vi "Voltage Sweep Merge.vi"() -> ()   [LabVIEW 2017]
doc: "This example shows how to create, run a script and query the script output data."
uses:
  <vilib>/Utility/file.llb/Write Delimited Spreadsheet (string).vi
  <instrlib>/Keithley 2600 Series/Keithley 2600 Series.lvlib
panel:
  out "Graph 3":T1(graph)
  in  "Working Folder":path=path "~"
  out "PCE(a.u.)":dbl
  in  "Pin(W/cm^2)":dbl=0.1
  out "FF(a.u.)":dbl
  out "Jsc(A/cm^2)":dbl
  in  "Area(cm^2)":dbl=0.085
  out "Ioc(A)":dbl
  out "Voc(V)":dbl
  out "Vsc(V)":dbl
  out "Isc(A)":dbl
  out "IMP(A)":dbl
  out "VMP(V)":dbl
  out "PMP(W)":dbl
  out "output array":string[][](array[string])
  in  "SweepSetting":T2={"CurrentLimit(A)"=0.1, "Start Voltage(V)"=-0.5, "Stop Voltage(V)"=0.9, "Dwell Time(mS)"=150.0, "NumPoint"=75.0} {"NumPoint" min=1.0 max=75.0 step=1.0; "Dwell Time(mS)" min=50.0 max=150.0; "Stop Voltage(V)" min=-200.0 max=200.0; "Start Voltage(V)" min=-200.0 max=200.0; "CurrentLimit(A)" min=1e-09 max=1.5}
  out "Graph 2":T1(graph)
  out "Sweep":i32
  in  "Inter Sweep Delay(s)":dbl=1.0 min=0.1 max=3600.0
  out "Seconds":i32
  out "Minutes":i32
  out "Hours":i32
  in  "Stop Button":bool
  in  "Aperture State (Channel B)":u16(ring) items=["Always OFF", "Always ON", "ON During Sweep OFF Otherwise", "OFF During Sweep ON Otherwise"]
  in  "Number of Sweeps":dbl=3.0 min=1.0 max=1000.0 step=1.0
  in  "USB COM Port":refnum<visa-resource-name>="COM3"
  # "Time Remaining"
  # ":"
  # ":"
  # "Sweep Setting\n(Channel A)"
  # "2634B can output up to 20.2 V at 1.5 A,\n or 202 V at 100 mA current limit."
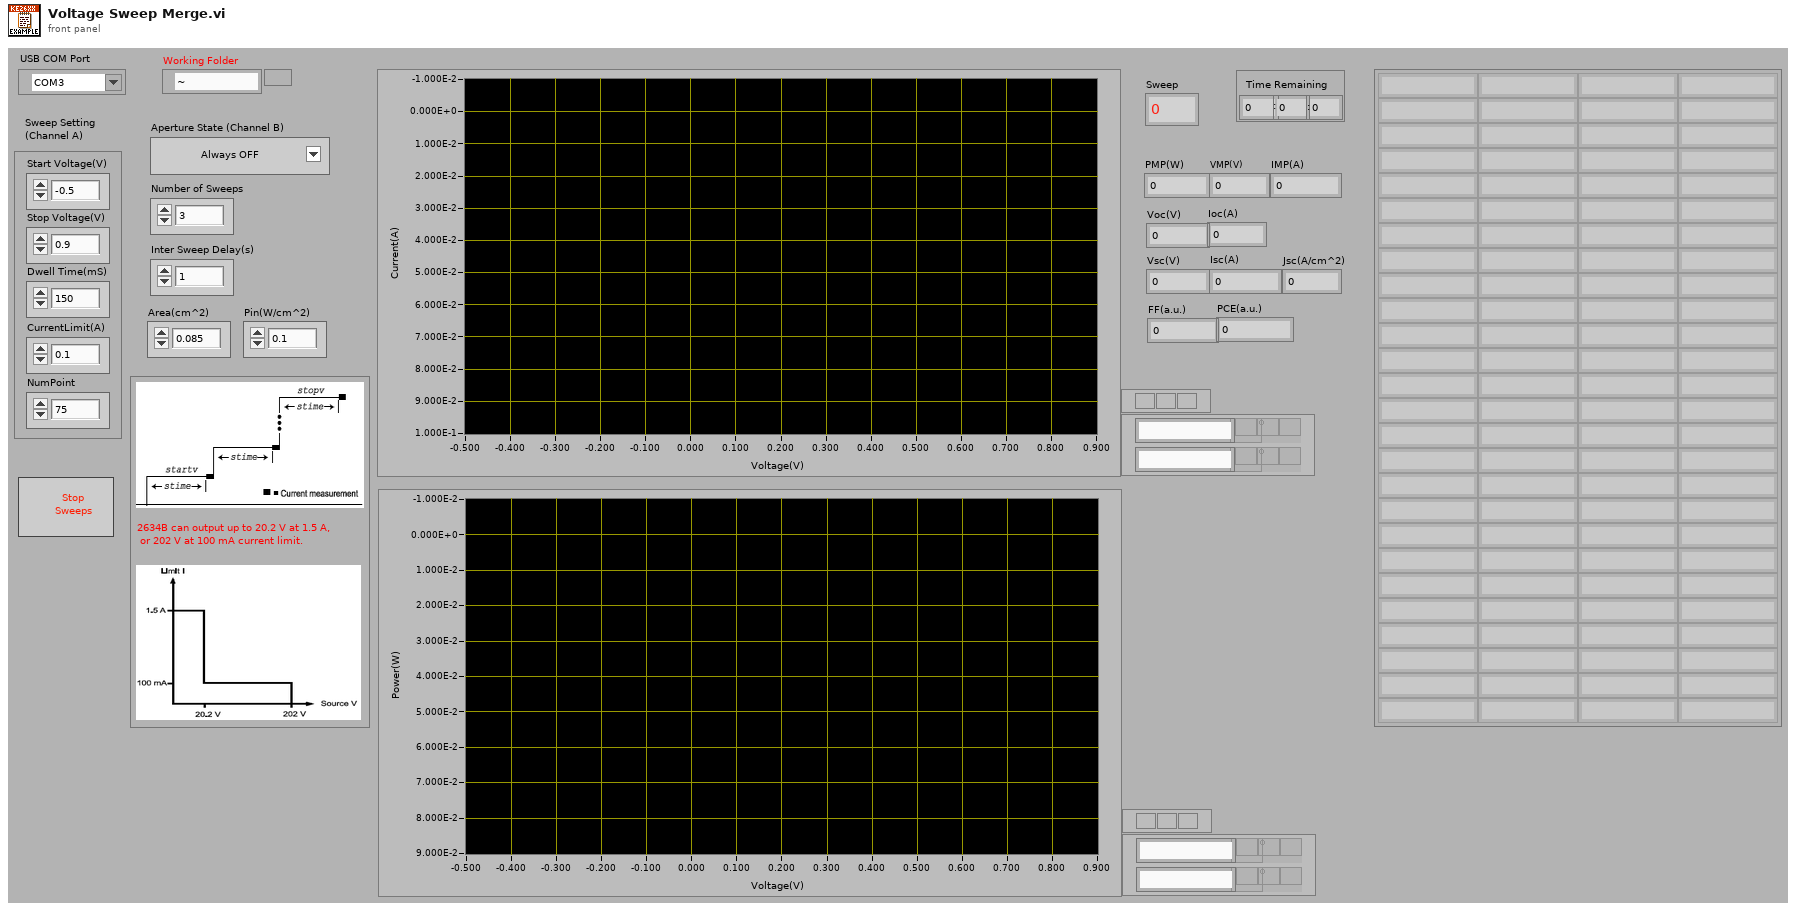
[diagram p1: front panel]
types:
  T1 = cluster{"array type (2D Dbl)":dbl[], "array type (2D Dbl)":dbl[]}
  T2 = cluster{"CurrentLimit(A)":dbl, "Start Voltage(V)":dbl, "Stop Voltage(V)":dbl, "Dwell Time(mS)":dbl, "NumPoint":dbl}
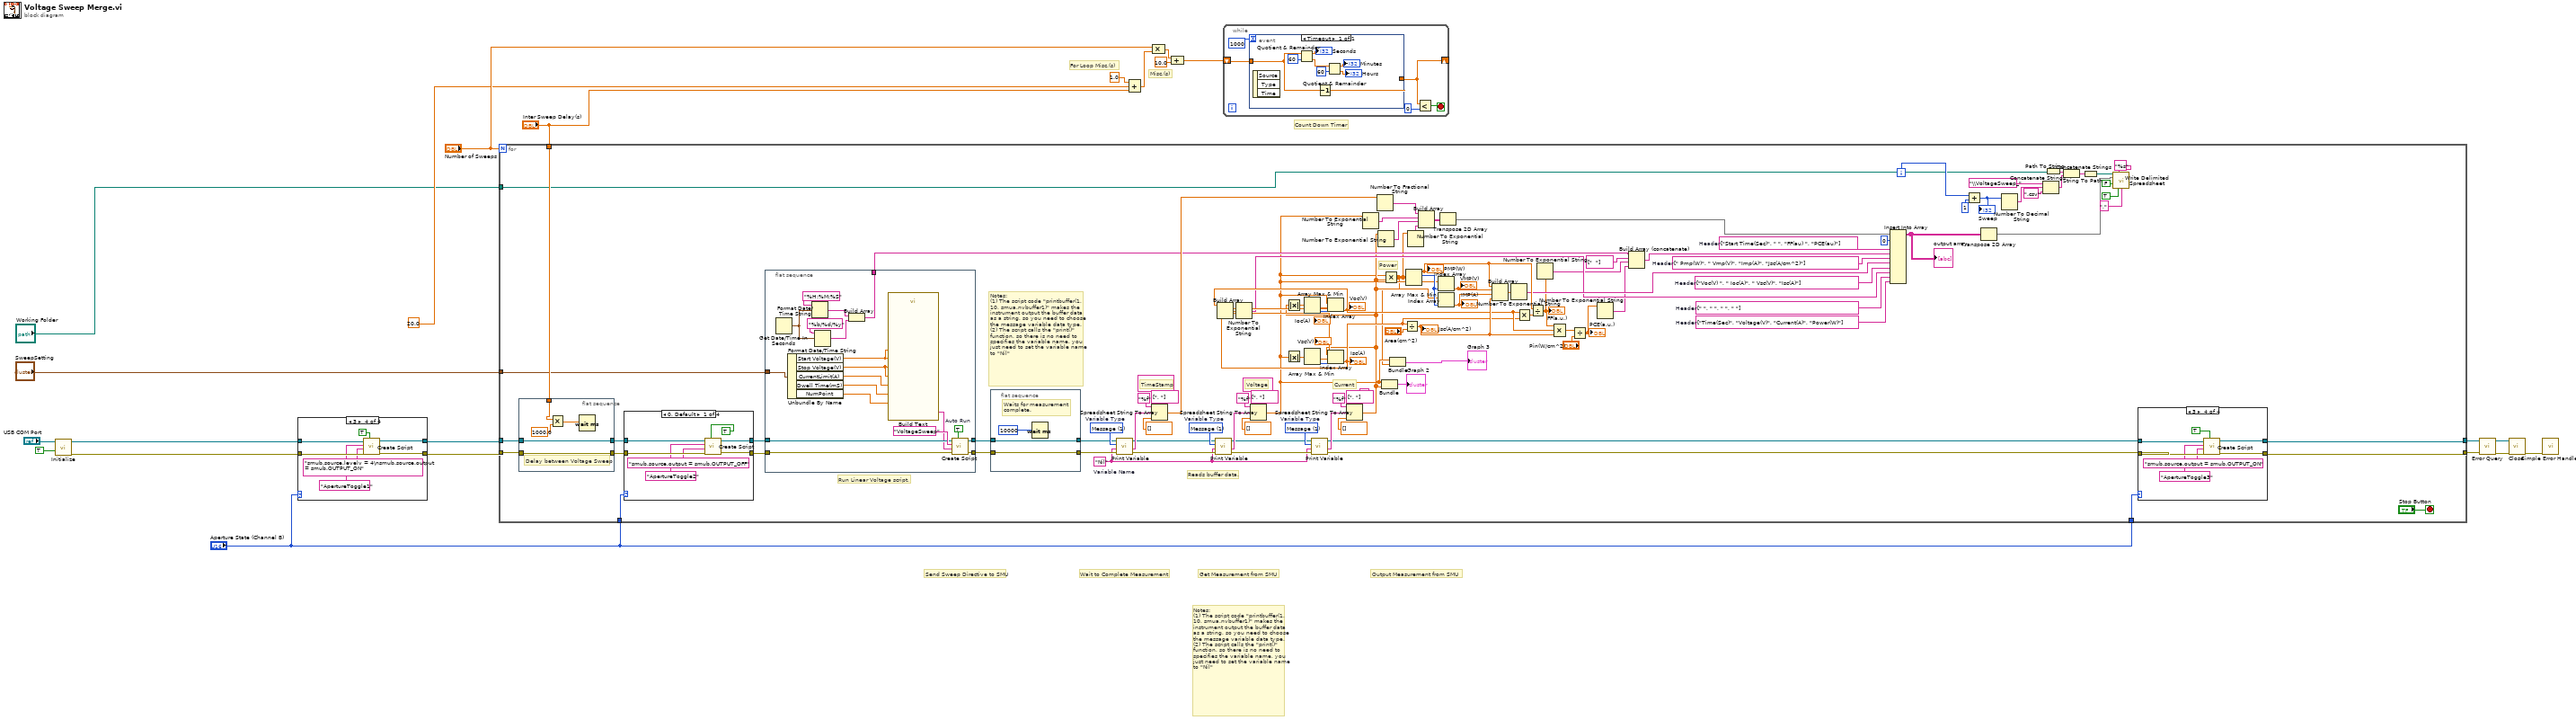
[diagram p0: block diagram]
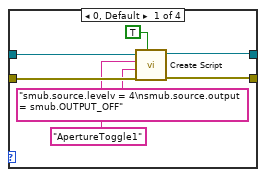
[diagram p2: hidden frame]
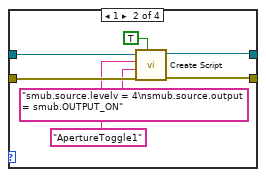
[diagram p3: hidden frame]
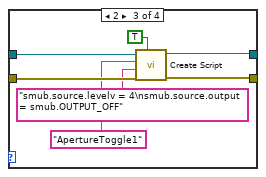
[diagram p4: hidden frame]
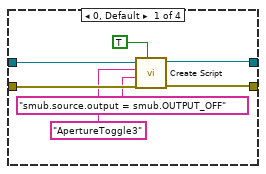
[diagram p5: hidden frame]
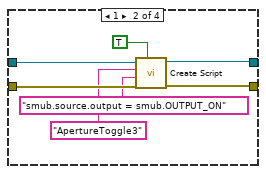
[diagram p6: hidden frame]
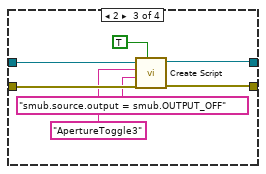
[diagram p7: hidden frame]
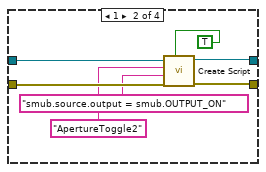
[diagram p8: hidden frame]
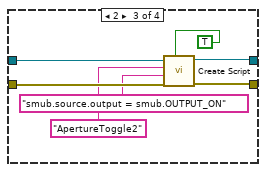
[diagram p9: hidden frame]
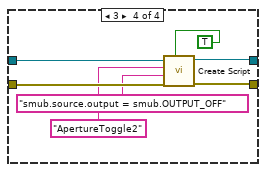
[diagram p10: hidden frame]
diagram:
  # "Count Down Timer"
  # "Misc.(s)"
  # "For Loop Misc.(s)"
  # "Send Sweep Directive to SMU"
  # "Wait to Complete Measurement"
  # "Output Measurement from SMU"
  # "Get Measurement from SMU"
  # "Notes: \n(1) The script code \"printbuffer(1, 10, smua.nvbuffer1)\" makes the instrument output the buffer data as a string, so you need to choose the message variable data type.\n(2) The script calls the \"print()\" function, so there is no need to specifies the variable name, you just need to set the variable name to \"Nil\""
  n1 = call <instrlib>:"Initialize.vi"("Reset (True)"=TRUE, "VISA resource name"="USB COM Port") -> ("error out"=w2:errorcluster, "VISA resource name out"=w14:refnum<visa-resource-name>)  [unwired: 8 in]
  n2 = case shown="3" "Aperture State (Channel B)" {
    tunnel: w14 -> [w29 w36 w43 w50]
    tunnel: w2 -> [w26 w33 w40 w47]
    tunnel: [w28 w35 w42 w49] -> w16
    tunnel: [w27 w34 w41 w48] -> w15
    frame 0, Default {
      n3 = call <instrlib>:"Create Script.vi"("Auto Run (F: Disable)"=TRUE, "error in (no error)"=w26, "Source Code"="smub.source.levelv = 4\nsmub.source.output = smub.OUTPUT_OFF", "Script Variable"="ApertureToggle1", "VISA resource name"=w29) -> ("error out"=w27:errorcluster, "VISA resource name out"=w28:refnum<visa-resource-name>)  [unwired: 5 in]
    }
    frame 1 {
      n4 = call <instrlib>:"Create Script.vi"("Auto Run (F: Disable)"=TRUE, "error in (no error)"=w33, "Source Code"="smub.source.levelv = 4\nsmub.source.output = smub.OUTPUT_ON", "Script Variable"="ApertureToggle1", "VISA resource name"=w36) -> ("error out"=w34:errorcluster, "VISA resource name out"=w35:refnum<visa-resource-name>)  [unwired: 5 in]
    }
    frame 2 {
      n5 = call <instrlib>:"Create Script.vi"("Auto Run (F: Disable)"=TRUE, "error in (no error)"=w40, "Source Code"="smub.source.levelv = 4\nsmub.source.output = smub.OUTPUT_OFF", "Script Variable"="ApertureToggle1", "VISA resource name"=w43) -> ("error out"=w41:errorcluster, "VISA resource name out"=w42:refnum<visa-resource-name>)  [unwired: 5 in]
    }
    frame 3 {
      n6 = call <instrlib>:"Create Script.vi"("Auto Run (F: Disable)"=TRUE, "error in (no error)"=w47, "Source Code"="smub.source.levelv = 4\nsmub.source.output = smub.OUTPUT_ON", "Script Variable"="ApertureToggle1", "VISA resource name"=w50) -> ("error out"=w48:errorcluster, "VISA resource name out"=w49:refnum<visa-resource-name>)  [unwired: 5 in]
    }
  }
  n7 = for {
    N: "Number of Sweeps" -> [_]
    tunnel: "Working Folder" -> [w66]
    tunnel: "Aperture State (Channel B)" -> [w148]
    tunnel: "Aperture State (Channel B)" -> [w147]
    tunnel: "Inter Sweep Delay(s)" -> [w146]
    tunnel: "SweepSetting" -> [w64]
    tunnel: w16 -> [w152]
    tunnel: [w52] -> w18
    tunnel: w15 -> [w151]
    tunnel: [w51] -> w17
    i -> [w132]
    stop <- "Stop Button" stop-if-true
    w74 = string[] ["Voc(V) ", " Ioc(A)", " Vsc(V)", "Isc(A)"]  # Header
    w75 = string[] [" Pmp(W)", " Vmp(V)", "Imp(A)", "Jsc(A/cm^2)"]  # Header
    w71 = string[] ["Time(Sec)", "Voltage(V)", "Current(A)", "Power(W)"]  # Header
    w72 = string[] [" ", " ", " ", " "]  # Header
    w88 = string[] ["Start Time(Sec)", " ", "FF(au) ", "PCE(au)"]  # Header
    w117 = 1 items=["Number", "Message"]  # Variable Type
    w118 = 1 items=["Number", "Message"]  # Variable Type
    w131 = 1 items=["Number", "Message"]  # Variable Type
    w108 = "Nil"  # Variable Name
    # "Power"
    # "Current"
    # "Voltage"
    # "TimeStamp"
    # "Reads buffer data."
    # "Notes: \n(1) The script code \"printbuffer(1, 10, smua.nvbuffer1)\" makes the instrument output the buffer data as a string, so you need to choose the message variable data type.\n(2) The script calls the \"print()\" function, so there is no need to specifies the variable name, you just need to set the variable name to \"Nil\""
    # "Run Linear Voltage script."
    n8 = flat-sequence {
      tunnel: w152 -> [w235]
      tunnel: w151 -> [w234]
      tunnel: [w235] -> w150
      tunnel: [w234] -> w149
      tunnel: w146 -> [w231]
      frame #0 {
        # "Delay between Voltage Sweep"
        n9 = Multiply(x=w231, y=1000.0) -> (x*y=w233:dbl)
        n10 = Wait (ms)(milliseconds to wait=w233) -> ()  [unwired: 1 out]
      }
    }
    n11 = case shown="0, Default" w148 {
      tunnel: w150 -> [w209 w216 w223 w230]
      tunnel: w149 -> [w206 w213 w220 w227]
      tunnel: [w208 w215 w222 w229] -> w70
      tunnel: [w207 w214 w221 w228] -> w69
      frame 0, Default {
        n12 = call <instrlib>:"Create Script.vi"("Auto Run (F: Disable)"=TRUE, "error in (no error)"=w206, "Source Code"="smub.source.output = smub.OUTPUT_OFF", "Script Variable"="ApertureToggle2", "VISA resource name"=w209) -> ("error out"=w207:errorcluster, "VISA resource name out"=w208:refnum<visa-resource-name>)  [unwired: 5 in]
      }
      frame 1 {
        n13 = call <instrlib>:"Create Script.vi"("Auto Run (F: Disable)"=TRUE, "error in (no error)"=w213, "Source Code"="smub.source.output = smub.OUTPUT_ON", "Script Variable"="ApertureToggle2", "VISA resource name"=w216) -> ("error out"=w214:errorcluster, "VISA resource name out"=w215:refnum<visa-resource-name>)  [unwired: 5 in]
      }
      frame 2 {
        n14 = call <instrlib>:"Create Script.vi"("Auto Run (F: Disable)"=TRUE, "error in (no error)"=w220, "Source Code"="smub.source.output = smub.OUTPUT_ON", "Script Variable"="ApertureToggle2", "VISA resource name"=w223) -> ("error out"=w221:errorcluster, "VISA resource name out"=w222:refnum<visa-resource-name>)  [unwired: 5 in]
      }
      frame 3 {
        n15 = call <instrlib>:"Create Script.vi"("Auto Run (F: Disable)"=TRUE, "error in (no error)"=w227, "Source Code"="smub.source.output = smub.OUTPUT_OFF", "Script Variable"="ApertureToggle2", "VISA resource name"=w230) -> ("error out"=w228:errorcluster, "VISA resource name out"=w229:refnum<visa-resource-name>)  [unwired: 5 in]
      }
    }
    n16 = flat-sequence {
      tunnel: [w169] -> w130
      tunnel: [w168] -> w129
      tunnel: w70 -> [w167]
      tunnel: w69 -> [w166]
      tunnel: [w159] -> w90
      tunnel: w64 -> [w153]
      frame #0 {
        w170 = TRUE  # Auto Run
        n17 = Get Date/Time In Seconds() -> (seconds since 1Jan1904=w160:timestamp)
        n18 = Unbundle By Name(w153) -> ("Start Voltage(V)"=w158:dbl, "Stop Voltage(V)"=w157:dbl, "CurrentLimit(A)"=w156:dbl, "Dwell Time(mS)"=w155:dbl, "NumPoint"=w154:dbl)
        n19 = Format Date/Time String(time format string (%c)="%H:%M:%S", seconds (now)=w160) -> (date/time string=w163:string)  [unwired: 1 out]
        n20 = Format Date/Time String(time format string (%c)="%b/%d/%y", seconds (now)=w160) -> (date/time string=w161:string)  [unwired: 1 out]
        n21 = Build Array(w163, w161) -> (w159:string[])
        n22 = call "Build Text"("numPoints"=w154, "stopV1"=w157, "limitI"=w156, "stopV"=w157, "startV"=w158, "startV1"=w158, "dwellTime"=w155) -> ("Result"=w165:string)  [unwired: 7 in, 1 out]
        n23 = call <instrlib>:"Create Script.vi"("Auto Run (F: Disable)"=w170, "error in (no error)"=w166, "Source Code"=w165, "Script Variable"="VoltageSweep" ("Script Variable (myScript)"), "VISA resource name"=w167) -> ("error out"=w168:errorcluster, "VISA resource name out"=w169:refnum<visa-resource-name>)  [unwired: 5 in]
      }
    }
    n24 = flat-sequence {
      tunnel: w130 -> [w172]
      tunnel: w129 -> [w173]
      tunnel: [w173] -> w127
      tunnel: [w172] -> w128
      frame #0 {
        # "Waits for measurement complete."
        n25 = Wait (ms)(milliseconds to wait=10000 ("Temp Delay")) -> ()  [unwired: 1 out]
      }
    }
    n26 = call <instrlib>:"Print Variable.vi"("error in (no error)"=w127, "Variable Name"=w108, "Variable Type (0: Number)"=w131, "VISA resource name"=w128) -> ("error out"=w114:errorcluster, "Message"=w123:string, "VISA resource name out"=w115:refnum<visa-resource-name>)  [unwired: 4 in, 1 out]
    n27 = Spreadsheet String To Array(delimiter (Tab)=string[] [", "], format string="%f", spreadsheet string=w123, array type (2D Dbl)=dbl[] []) -> (array=w103:dbl[])
    n28 = call <instrlib>:"Print Variable.vi"("error in (no error)"=w114, "Variable Name"=w108, "Variable Type (0: Number)"=w118, "VISA resource name"=w115) -> ("error out"=w112:errorcluster, "Message"=w122:string, "VISA resource name out"=w113:refnum<visa-resource-name>)  [unwired: 4 in, 1 out]
    n29 = Spreadsheet String To Array(delimiter (Tab)=string[] [", "], format string="%f", spreadsheet string=w122, array type (2D Dbl)=dbl[] []) -> (array=w54:dbl[])
    n30 = Absolute Value(x=w54) -> (abs(x)=w99:dbl[])
    n31 = Array Max & Min(array=w99) -> (min value=w77:dbl, min index (indices)=w98:i32)  [unwired: 2 out]
    "Vsc(V)" <- w77
    n32 = call <instrlib>:"Print Variable.vi"("error in (no error)"=w112, "Variable Name"=w108, "Variable Type (0: Number)"=w117, "VISA resource name"=w113) -> ("error out"=w67:errorcluster, "Message"=w110:string, "VISA resource name out"=w68:refnum<visa-resource-name>)  [unwired: 4 in, 1 out]
    n33 = Spreadsheet String To Array(delimiter (Tab)=string[] [", "], format string="%f", spreadsheet string=w110, array type (2D Dbl)=dbl[] []) -> (array=w57:dbl[])
    n34 = Absolute Value(x=w57) -> (abs(x)=w96:dbl[])
    n35 = Array Max & Min(array=w96) -> (min value=w78:dbl, min index (indices)=w97:i32)  [unwired: 2 out]
    "Ioc(A)" <- w78
    n36 = Index Array(array=w54, index=w97) -> (element=w79:dbl)
    "Voc(V)" <- w79
    n37 = Index Array(array=w57, index=w98) -> (element=w76:dbl)
    "Isc(A)" <- w76
    n38 = Build Array(w79, w78, w77, w76) -> (w80:dbl[])
    n39 = Number To Exponential String(number=w80) -> (E-format string=w73:string[])  [unwired: 3 in]
    n40 = Number To Exponential String(number=w54) -> (E-format string=w105:string[])  [unwired: 3 in]
    n41 = Number To Fractional String(number=w103) -> (F-format string=w106:string[])  [unwired: 3 in]
    n42 = Number To Exponential String(number=w57) -> (E-format string=w101:string[])  [unwired: 3 in]
    n43 = Bundle("array type (2D Dbl)"=w54, "array type (2D Dbl)"=w57) -> (→"Graph 2":T1)  [unwired: 1 in]
    n44 = Multiply(x=w54, y=w57) -> (x*y=w53:dbl[])
    n45 = Bundle("array type (2D Dbl)"=w54, w53) -> (→"Graph 3":cluster{"array type (2D Dbl)":dbl[], dbl[]})  [unwired: 1 in]
    n46 = Divide(x=w76, y="Area(cm^2)") -> (x/y=w83:dbl)
    "Jsc(A/cm^2)" <- w83
    n47 = Array Max & Min(array=w53) -> (max value=w86:dbl, max index (indices)=w100:i32)  [unwired: 2 out]
    "PMP(W)" <- w86
    n48 = Number To Exponential String(number=w53) -> (E-format string=w91:string[])  [unwired: 3 in]
    n49 = Build Array(w106, w105, w101, w91) -> (w107:string[][])
    n50 = Index Array(array=w54, index=w100) -> (element=w85:dbl)
    "VMP(V)" <- w85
    n51 = Index Array(array=w57, index=w100) -> (element=w84:dbl)
    "IMP(A)" <- w84
    n52 = Transpose 2D Array(2D array=w107) -> (transposed array=w104:string[][])
    n53 = Build Array(w86, w85, w84, w83) -> (w82:dbl[])
    n54 = Number To Exponential String(number=w82) -> (E-format string=w81:string[])  [unwired: 3 in]
    n55 = Multiply(x=w76, y=w79) -> (x*y=w94:dbl)
    n56 = Divide(x=w86, y=w94) -> (x/y=w63:dbl)
    "FF(a.u.)" <- w63
    n57 = Number To Exponential String(number=w63) -> (E-format string=w62:string)  [unwired: 3 in]
    n58 = Compound Arithmetic op=MULTIPLY(w63, w79, w83) -> (w93:dbl)
    n59 = Divide(x=w93, y="Pin(W/cm^2)") -> (x/y=w61:dbl)
    "PCE(a.u.)" <- w61
    n60 = Number To Exponential String(number=w61) -> (E-format string=w60:string)  [unwired: 3 in]
    n61 = Build Array (concatenate)(w90, string[] ["  "] ("element"), w62, w60) -> (w87:string[])
    n62 = Insert Into Array(array=w104, index (row)=0, new element #1=w88, new element #2=w87, new element #3=w75, new element #4=w81, new element #5=w74, new element #6=w73, new element #7=w72, new element #8=w71) -> (w65:string[][])  [unwired: 1 in]
    "output array" <- w65
    n63 = Add(x=w132, y=1 ("x")) -> (x+y=w145:i32)
    "Sweep" <- w145
    n64 = Transpose 2D Array(2D array=w65) -> (transposed array=w59:string[][])
    n65 = Number To Decimal String(number=w145) -> (decimal integer string=w144:string)  [unwired: 1 in]
    n66 = Concatenate Strings("\\VoltageSweep_" ("string"), w144, ".csv" ("string")) -> (w143:string)
    n67 = Path To String(path=w66) -> (string=w140:string)
    n68 = Concatenate Strings(w140, w143) -> (w141:string)
    n69 = String To Path(string=w141) -> (path=w142:path)
    n70 = call-poly <vilib>:"Write Delimited Spreadsheet.vi"("file path (dialog if empty)"=w142, "format (%s)"="%s" ("format (%.3f)"), "2D data"=w59, "append to file? (new file:F)"=FALSE, "transpose? (no:F)"=TRUE, "delimiter (\\t)"="," ("delimiter (\\t)")) -> ()  [unwired: 8 in, 2 out]
    n71 = case shown="3" w147 {
      tunnel: w68 -> [w181 w188 w195 w202]
      tunnel: w67 -> [w178 w185 w192 w199]
      tunnel: [w180 w187 w194 w201] -> w52
      tunnel: [w179 w186 w193 w200] -> w51
      frame 0, Default {
        n72 = call <instrlib>:"Create Script.vi"("Auto Run (F: Disable)"=TRUE, "error in (no error)"=w178, "Source Code"="smub.source.output = smub.OUTPUT_OFF", "Script Variable"="ApertureToggle3", "VISA resource name"=w181) -> ("error out"=w179:errorcluster, "VISA resource name out"=w180:refnum<visa-resource-name>)  [unwired: 5 in]
      }
      frame 1 {
        n73 = call <instrlib>:"Create Script.vi"("Auto Run (F: Disable)"=TRUE, "error in (no error)"=w185, "Source Code"="smub.source.output = smub.OUTPUT_ON", "Script Variable"="ApertureToggle3", "VISA resource name"=w188) -> ("error out"=w186:errorcluster, "VISA resource name out"=w187:refnum<visa-resource-name>)  [unwired: 5 in]
      }
      frame 2 {
        n74 = call <instrlib>:"Create Script.vi"("Auto Run (F: Disable)"=TRUE, "error in (no error)"=w192, "Source Code"="smub.source.output = smub.OUTPUT_OFF", "Script Variable"="ApertureToggle3", "VISA resource name"=w195) -> ("error out"=w193:errorcluster, "VISA resource name out"=w194:refnum<visa-resource-name>)  [unwired: 5 in]
      }
      frame 3 {
        n75 = call <instrlib>:"Create Script.vi"("Auto Run (F: Disable)"=TRUE, "error in (no error)"=w199, "Source Code"="smub.source.output = smub.OUTPUT_ON", "Script Variable"="ApertureToggle3", "VISA resource name"=w202) -> ("error out"=w200:errorcluster, "VISA resource name out"=w201:refnum<visa-resource-name>)  [unwired: 5 in]
      }
    }
  }
  n76 = Compound Arithmetic op=ADD(1.0 ("value"), 20.0 ("value"), "Inter Sweep Delay(s)") -> (w11:dbl)
  n77 = Compound Arithmetic op=MULTIPLY("Number of Sweeps", w11) -> (w10:dbl)
  n78 = Compound Arithmetic op=ADD(w10, 10.0 ("value")) -> (w8:dbl)
  n79 = while {
    shift-right: [w237] -> _
    shift-left: w8 -> [w239]
    stop <- w238 stop-if-true
    n80 = event shown="[0] Timeout" {
      selector: _ -> [_]
      dyn-events: _ -> [_]
      timeout: 1000 -> [_]
      tunnel: w239 -> [w246]
      tunnel: [w248] -> w237
      event Timeout {
        n81 = event-data() -> ()  [unwired: 1 in, 3 out]
        n82 = Quotient & Remainder(x=w246, y=60) -> (x-y*floor(x/y)=→"Seconds":dbl, floor(x/y)=w242:dbl)
        n83 = Decrement(x=w246) -> (x-1=w248:dbl)
        n84 = Quotient & Remainder(x=w242, y=60) -> (x-y*floor(x/y)=→"Minutes":dbl, floor(x/y)=→"Hours":dbl)
      }
    }
    n85 = Less?(x=w237, y=0) -> (x < y?=w238:bool)
  }
  n86 = call <instrlib>:"Error Query.vi"("error in (no error)"=w17, "VISA resource name"=w18) -> ("error out"=w21:errorcluster, "VISA resource name out"=w22:refnum<visa-resource-name>)  [unwired: 6 in, 2 out]
  n87 = call <instrlib>:"Close.vi"("error in (no error)"=w21, "VISA resource name"=w22) -> ("error out"=w4:errorcluster)  [unwired: 9 in]
  n88 = call <vilib>:"Simple Error Handler.vi"("error in (no error)"=w4) -> ()  [unwired: 4 in, 5 out]
